vi "z go delay.vi"(8 "Delay Time (s)":dbl=1.0, 9 "Speed":dbl=5.0 format="%#_13g", 10 "Position":dbl=30.0 format="%#_13g", 11 "Motion.lvclass":refnum<class "Motion.lvclass">) -> (3 "Motion.lvclass 2":refnum<class "Motion.lvclass">)   [LabVIEW 2016]
uses:
  Classes/Controller/Motion/Motion Folder/Motion.lvclass
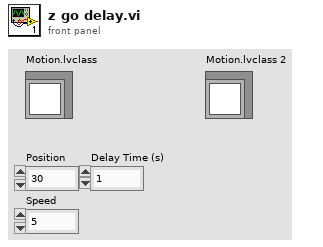
[diagram p1: front panel]
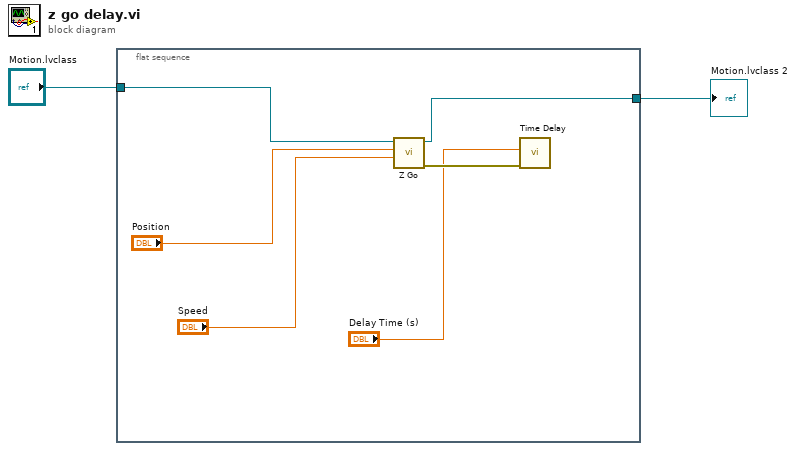
[diagram p0: block diagram]
diagram:
  n1 = flat-sequence {
    tunnel: [w7] -> w2
    tunnel: "Motion.lvclass" -> [w6]
    frame #0 {
      n2 = call-dynamic "Z Go.vi"("Speed"="Speed", "Position"="Position", "Motion in"=w6) -> ("error out"=w8:errorcluster, "Motion out"=w7:refnum<class "Motion.lvclass">)  [unwired: 7 in]
      n3 = call "Time Delay"("error in (no error)"=w8, "Delay Time (s)"="Delay Time (s)") -> ()  [unwired: 9 in, 1 out]
    }
  }
  "Motion.lvclass 2" <- w2
